vi "Read Pressure.vi"(8 "error in (no error)":errorcluster, 11 "Pressure Actor.lvlib:Pressure.lvclass":refnum<class "Pressure.lvclass">) -> (0 "error out":errorcluster, 3 "Actor out":refnum<class "Actor.lvclass">)   [LabVIEW 2018, in "Pressure Actor.lvlib" / "Pressure.lvclass"]
uses:
  Pressure.lvclass
  C:/Program Files (x86)/National Instruments/LabVIEW 2018/vi.lib/ActorFramework/Actor/Actor.lvclass
  <vilib>/ActorFramework/Actor/Actor.lvclass
  Pressure.lvclass/Pressure.ctl
  <vilib>/DAQmx/read.llb/DAQmx Read (Analog DBL 1Chan 1Samp).vi
  <vilib>/DAQmx/miscellaneous.llb/DAQmx Fill In Error Info.vi
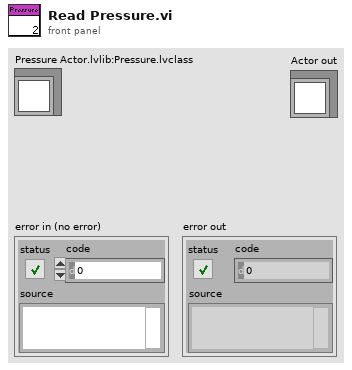
[diagram p1: front panel]
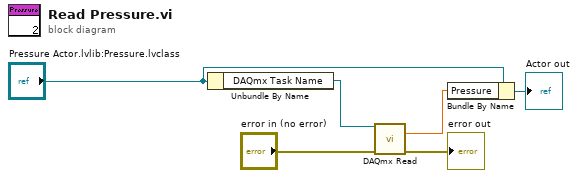
[diagram p0: block diagram]
diagram:
  n1 = Unbundle By Name("Pressure Actor.lvlib:Pressure.lvclass") -> ("DAQmx Task Name"=w6:refnum<k21>)
  n2 = call-poly <vilib>:"DAQmx Read.vi"("task/channels in"=w6, "error in"="error in (no error)") -> ("data"=w2:dbl, "error out"=→"error out":errorcluster)  [unwired: 11 in, 1 out]
  n3 = Bundle By Name(cluster="Pressure Actor.lvlib:Pressure.lvclass", "Pressure"=w2) -> (→"Actor out":refnum<class "Pressure.lvclass">)
